vi "Read Histogram Averages.vi"(8 "error in (no error)":errorcluster, 11 "VISA resource name":refnum<visa-resource-name>) -> (0 "error out":errorcluster, 1 "Histogram Median":dbl, 2 "Histogram Mean":dbl, 3 "VISA resource name out":refnum<visa-resource-name>, 5 "Histogram Mode":dbl)   [LabVIEW 2016, in "Agilent 2000 3000 X-Series.lvlib"]
doc: "Returns the averages of number of hits on the histogram.\n\n<b>Note:</b>\nThis VI is specific to the 6000-X Series oscilloscopes. These features are not available on other models."
uses:
  Agilent 2000 3000 X-Series.lvlib
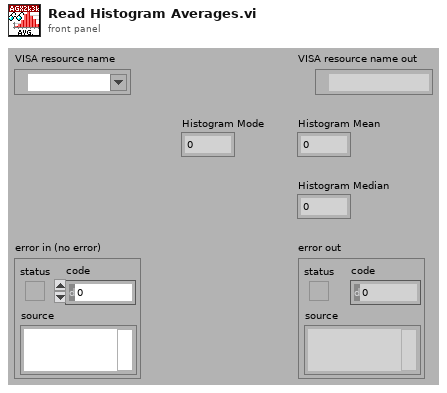
[diagram p1: front panel]
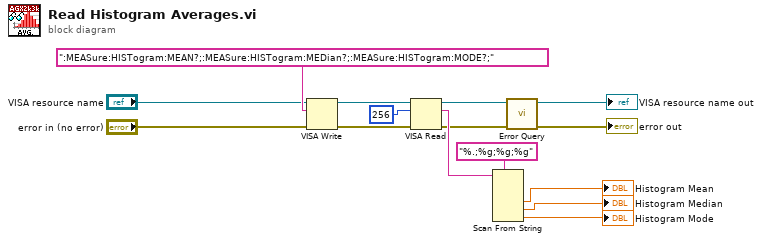
[diagram p0: block diagram]
diagram:
  n1 = VISA Write(VISA resource name="VISA resource name", write buffer=":MEASure:HISTogram:MEAN?;:MEASure:HISTogram:MEDian?;:MEASure:HISTogram:MODE?;", error in (no error)="error in (no error)") -> (VISA resource name out=w8:refnum<visa-resource-name>, error out=w9:errorcluster)  [unwired: 1 out]
  n2 = VISA Read(VISA resource name=w8, byte count=u32 256, error in (no error)=w9) -> (VISA resource name out=w4:refnum<visa-resource-name>, read buffer=w12:string, error out=w3:errorcluster)  [unwired: 1 out]
  n3 = Scan From String(format string="%.;%g;%g;%g", input string=w12) -> (output 1=→"Histogram Mean":dbl, output 2=→"Histogram Median":dbl, output 3=→"Histogram Mode":dbl)  [unwired: 5 in, 3 out]
  n4 = call "Error Query.vi"("error in (no error)"=w3, "VISA resource name"=w4) -> ("error out"=→"error out":errorcluster, "VISA resource name out"=→"VISA resource name out":refnum<visa-resource-name>)  [unwired: 6 in, 2 out]
